vi "3_2_MNIST_Inference(FPGA)(PXI).vi"() -> ()   [LabVIEW 2020]
uses:
  <vilib>/userDefined/High Color/nirio_resource_hc.ctl
  <vilib>/Ngene/DeepLTK FPGA Addon/Toolkit/NNF_Host/Low_Level/NNF_Init/Controls/NNF_FPGA_Target_Info.ctl
  <extravilib>/ChannelInstances/Tag-bool/Write With Abort.vi
  <extravilib>/ChannelInstances/Tag-bool/Read With Abort.vi
  <extravilib>/ChannelInstances/Tag-bool/Instantiate.vi
  <vilib>/FPGAPlugInAG/Dynamic/niLvFpga_Download_Dynamic.vi
  <vilib>/FPGAPlugInAG/Dynamic/niLvFpga_Run_Dynamic.vi
  <extravilib>/ChannelInstances/Tag-bool/EndpointRead.vi
  <vilib>/Ngene/DeepLTK FPGA Addon/Toolkit/NNF_Host/API/NNF_Set_Input/NNF_Set_Input(2D_I8).vi
  <vilib>/FPGAPlugInAG/Dynamic/niLvFpga_Close_Dynamic.vi
  <extravilib>/ChannelInstances/Tag-bool/Endpoint.vi
  <vilib>/rvi/interface/nirviMethod/nirviMethod.xnode
  <vilib>/rvi/interface/nirviCloseFPGA/nirviCloseFPGA.xnode
  <extravilib>/ChannelInstances/Tag-bool.lvlib
  <vilib>/Ngene/DeepLTK FPGA Addon/Toolkit/DeepLTK_FPGA_Addon.lvlib
  <vilib>/Ngene/Deep Learning Toolkit/Toolkit/Deep_Learning_Toolkit_by_Ngene.lvlib
  <vilib>/ptbypt/NI_PtbyPt.lvlib
panel:
  out "Target Information":T1={"BRAM _Buff_1_Size"=52500, "BRAM _Buff_2_Size"=45937, "Version"=[8, 1, 1, 0], "# Cores"=8}
  out "Predictions":sgl[](array[slide])=[5.797983e-07, 2.833721e-05, 6.34908e-06, 0.999726, 5.797983e-07, 6.952559e-05, 3.4902146e-06, 1.1549668e-05, 9.3772185e-05, 5.9866026e-05] scale=0.0..1.0
  out "test time(s/img)":dbl=0.014425458999976399 format="%#_3p"
  out "Test Speed (img/s)":dbl=69.32188431589151 format="%#_3p"
  in  "FPGA Bitfile":path=path "D:/Ngene/GitHub/deepltk_fpga_examples/FPGA Bitfiles/NNF_sbRIO_9609_8Cores.lvbitx"
  in  "FPGA Target":T2="rio://10.0.0.39/RIO0" caption="RIO Device"
  in  "Weight File Path":path=path "D:/Ngene/GitHub/deepltk_fpga_examples/1_MNIST_Classification(PXI,sbRIO)/Models/1_Converted/mnist_cnn/NNF_mnist_cnn_weights_24_11_25__15_36_06.bin"
  in  "Configuration File Path":path=path "D:/Ngene/GitHub/deepltk_fpga_examples/1_MNIST_Classification(PXI,sbRIO)/Models/1_Converted/mnist_cnn/NNF_mnist_cnn_net_cfg_24_11_25__15_36_06.cfg"
  in  "Scalers File Path":path=path "D:/Ngene/GitHub/deepltk_fpga_examples/1_MNIST_Classification(PXI,sbRIO)/Models/1_Converted/mnist_cnn/NNF_mnist_cnn_net_scalers_24_11_25__15_36_06.cfg"
  out "Labels":string[](array[string])=["0", "1", "2", "3", "4", "5", "6", "7", "8", "9"]
  out "Pen Attributes":T3={"Width"=24, "Style"=enum."Solid"}
  out "Draw Digit (280x280 px)":picture
  in  "Pen Color":u32(colorbox)=197379
  in  "Stop":bool
  in  "Pen Width":dbl=24.0
  in  "Stop":bool
  out "image (28x28px)":sgl[][](graph)=[[-1.0, -1.0, -1.0, -1.0, -1.0, -1.0, -1.0, -1.0, -1.0, -1.0, -1.0, -1.0, -1.0, -1.0, -1.0, -1.0, -1.0, -1.0, -1.0, -1.0, -1.0, -1.0, -1.0, -1.0, -1.0, -1.0, -1.0, -1.0], [-1.0, -1.0, -1.0, -1.0, -1.0, -1.0, -1.0, -1.0, -1.0, -1.0, -1.0, -1.0, -1.0, -1.0, -1.0, -1.0, -1.0, -1.0, -1.0, -1.0, -1.0, -1.0, -1.0, -1.0, -1.0, -1.0, -1.0, -1.0], [-1.0, -1.0, -1.0, -1.0, -1.0, -1.0, -1.0, -0.96015626, -0.56171876, -0.1234375, 0.17539063, 0.49414062, 0.59375, 0.59375, 0.59375, 0.41445312, -0.08359375, -0.96015626, -1.0, -1.0, -1.0, -1.0, -1.0, -1.0, -1.0, -1.0, -1.0, -1.0], [-1.0, -1.0, -1.0, -1.0, -1.0, -0.9003906, 0.055859376, 0.8527344, 0.9921875, 0.9921875, 0.9921875, 0.9921875, 0.9921875, 0.9921875, 0.9921875, 0.9921875, 0.9921875, 0.6734375, -0.80078125, -1.0, -1.0, -1.0, -1.0, -1.0, -1.0, -1.0, -1.0, -1.0], [-1.0, -1.0, -1.0, -1.0, -0.840625, 0.77304685, 0.9921875, 0.9921875, 0.9921875, 0.9125, 0.6136719, 0.29492188, 0.1953125, 0.1953125, 0.1953125, 0.5738281, 0.9921875, 0.9921875, 0.17539063, -1.0, -1.0, -1.0, -1.0, -1.0, -1.0, -1.0, -1.0, -1.0], [-1.0, -1.0, -1.0, -1.0, -0.5816406, 0.9921875, 0.9921875, 0.37460938, -0.521875, -0.9800781, -1.0, -1.0, -1.0, -1.0, -1.0, -1.0, 0.7132813, 0.9921875, 0.31484374, -1.0, -1.0, -1.0, -1.0, -1.0, -1.0, -1.0, -1.0, -1.0], [-1.0, -1.0, -1.0, -1.0, -1.0, -0.22304687, -0.22304687, -1.0, -1.0, -1.0, -1.0, -1.0, -1.0, -1.0, -1.0, 0.095703125, 0.9921875, 0.9921875, 0.055859376, -1.0, -1.0, -1.0, -1.0, -1.0, -1.0, -1.0, -1.0, -1.0], [-1.0, -1.0, -1.0, -1.0, -1.0, -1.0, -1.0, -1.0, -1.0, -1.0, -1.0, -1.0, -1.0, -1.0, 0.095703125, 0.9921875, 0.9921875, 0.63359374, -0.80078125, -1.0, -1.0, -1.0, -1.0, -1.0, -1.0, -1.0, -1.0, -1.0], [-1.0, -1.0, -1.0, -1.0, -1.0, -1.0, -1.0, -1.0, -1.0, -1.0, -1.0, -1.0, -1.0, 0.095703125, 0.9921875, 0.9921875, 0.6734375, -0.80078125, -1.0, -1.0, -1.0, -1.0, -1.0, -1.0, -1.0, -1.0, -1.0, -1.0], [-1.0, -1.0, -1.0, -1.0, -1.0, -1.0, -1.0, -1.0, -1.0, -1.0, -1.0, -0.9203125, 0.37460938, 0.9921875, 0.9921875, 0.65351564, -0.80078125, -1.0, -1.0, -1.0, -1.0, -1.0, -1.0, -1.0, -1.0, -1.0, -1.0, -1.0], [-1.0, -1.0, -1.0, -1.0, -1.0, -1.0, -1.0, -1.0, -1.0, -0.68125, -0.1234375, 0.7332031, 0.9921875, 0.9921875, 0.9921875, 0.6734375, -0.14335938, -1.0, -1.0, -1.0, -1.0, -1.0, -1.0, -1.0, -1.0, -1.0, -1.0, -1.0], [-1.0, -1.0, -1.0, -1.0, -1.0, -1.0, -1.0, -1.0, 0.0359375, 0.9921875, 0.9921875, 0.9921875, 0.9921875, 0.9921875, 0.9921875, 0.9921875, 0.9921875, -0.023828125, -1.0, -1.0, -1.0, -1.0, -1.0, -1.0, -1.0, -1.0, -1.0, -1.0], [-1.0, -1.0, -1.0, -1.0, -1.0, -1.0, -1.0, -1.0, 0.753125, 0.9921875, 0.9921875, 0.79296875, 0.25507814, 0.055859376, 0.1953125, 0.7132813, 0.9921875, 0.8925781, -0.9003906, -1.0, -1.0, -1.0, -1.0, -1.0, -1.0, -1.0, -1.0, -1.0], [-1.0, -1.0, -1.0, -1.0, -1.0, -1.0, -1.0, -1.0, -0.521875, -0.00390625, -0.42226562, -0.9800781, -1.0, -1.0, -1.0, -0.16328125, 0.9921875, 0.9921875, -0.9203125, -1.0, -1.0, -1.0, -1.0, -1.0, -1.0, -1.0, -1.0, -1.0], [-1.0, -1.0, -1.0, -1.0, -1.0, -1.0, -1.0, -1.0, -1.0, -1.0, -1.0, -1.0, -1.0, -1.0, -1.0, -0.1234375, 0.9921875, 0.9921875, -1.0, -1.0, -1.0, -1.0, -1.0, -1.0, -1.0, -1.0, -1.0, -1.0], [-1.0, -1.0, -1.0, -1.0, -1.0, -1.0, -1.0, -1.0, -1.0, -1.0, -1.0, -1.0, -1.0, -1.0, -0.7609375, 0.8527344, 0.9921875, 0.79296875, -1.0, -1.0, -1.0, -1.0, -1.0, -1.0, -1.0, -1.0, -1.0, -1.0], [-1.0, -1.0, -1.0, -1.0, -1.0, -1.0, -1.0, -1.0, -1.0, -1.0, -1.0, -1.0, -1.0, -0.80078125, 0.6933594, 0.9921875, 0.9722656, -0.40234375, -1.0, -1.0, -1.0, -1.0, -1.0, -1.0, -1.0, -1.0, -1.0, -1.0], [-1.0, -1.0, -1.0, -1.0, -1.0, -1.0, -1.0, -1.0, -1.0, -1.0, -1.0, -1.0, -0.7210938, 0.6933594, 0.9921875, 0.9921875, -0.06367187, -1.0, -1.0, -1.0, -1.0, -1.0, -1.0, -1.0, -1.0, -1.0, -1.0, -1.0], [-1.0, -1.0, -1.0, -1.0, -1.0, -1.0, -1.0, -1.0, -1.0, -1.0, -0.9003906, -0.22304687, 0.8726562, 0.9921875, 0.9921875, 0.095703125, -1.0, -1.0, -1.0, -1.0, -1.0, -1.0, -1.0, -1.0, -1.0, -1.0, -1.0, -1.0], [-1.0, -1.0, -0.9800781, 0.275, 0.79296875, 0.79296875, 0.79296875, 0.79296875, 0.79296875, 0.8726562, 0.9921875, 0.9921875, 0.9921875, 0.9722656, -0.023828125, -1.0, -1.0, -1.0, -1.0, -1.0, -1.0, -1.0, -1.0, -1.0, -1.0, -1.0, -1.0, -1.0], [-1.0, -1.0, -0.840625, 0.9921875, 0.9921875, 0.9921875, 0.9921875, 0.9921875, 0.9921875, 0.9921875, 0.9921875, 0.9921875, 0.7332031, -0.6015625, -1.0, -1.0, -1.0, -1.0, -1.0, -1.0, -1.0, -1.0, -1.0, -1.0, -1.0, -1.0, -1.0, -1.0], [-1.0, -1.0, -1.0, -0.2828125, 0.17539063, 0.13554688, 0.0359375, 0.1953125, 0.095703125, -0.00390625, -0.203125, -0.6015625, -0.96015626, -1.0, -1.0, -1.0, -1.0, -1.0, -1.0, -1.0, -1.0, -1.0, -1.0, -1.0, -1.0, -1.0, -1.0, -1.0], [-1.0, -1.0, -1.0, -1.0, -1.0, -1.0, -1.0, -1.0, -1.0, -1.0, -1.0, -1.0, -1.0, -1.0, -1.0, -1.0, -1.0, -1.0, -1.0, -1.0, -1.0, -1.0, -1.0, -1.0, -1.0, -1.0, -1.0, -1.0], [-1.0, -1.0, -1.0, -1.0, -1.0, -1.0, -1.0, -1.0, -1.0, -1.0, -1.0, -1.0, -1.0, -1.0, -1.0, -1.0, -1.0, -1.0, -1.0, -1.0, -1.0, -1.0, -1.0, -1.0, -1.0, -1.0, -1.0, -1.0], [-1.0, -1.0, -1.0, -1.0, -1.0, -1.0, -1.0, -1.0, -1.0, -1.0, -1.0, -1.0, -1.0, -1.0, -1.0, -1.0, -1.0, -1.0, -1.0, -1.0, -1.0, -1.0, -1.0, -1.0, -1.0, -1.0, -1.0, -1.0], [-1.0, -1.0, -1.0, -1.0, -1.0, -1.0, -1.0, -1.0, -1.0, -1.0, -1.0, -1.0, -1.0, -1.0, -1.0, -1.0, -1.0, -1.0, -1.0, -1.0, -1.0, -1.0, -1.0, -1.0, -1.0, -1.0, -1.0, -1.0], [-1.0, -1.0, -1.0, -1.0, -1.0, -1.0, -1.0, -1.0, -1.0, -1.0, -1.0, -1.0, -1.0, -1.0, -1.0, -1.0, -1.0, -1.0, -1.0, -1.0, -1.0, -1.0, -1.0, -1.0, -1.0, -1.0, -1.0, -1.0], [-1.0, -1.0, -1.0, -1.0, -1.0, -1.0, -1.0, -1.0, -1.0, -1.0, -1.0, -1.0, -1.0, -1.0, -1.0, -1.0, -1.0, -1.0, -1.0, -1.0, -1.0, -1.0, -1.0, -1.0, -1.0, -1.0, -1.0, -1.0]]
  # "Overview: Demonstrates the usage of DeepLTK FPGA Addon for loading the model pretrained for MNIST Classification and running for inference on FPGA Targets in PXI sytems.\nRequirements:\n•DeepLTK - Deep Learning Toolkit for LabVIEW (https://www.ngene.co/deep-learning-toolkit-for-labview)\n•DeepLTK FPGA Addon (https://www.ngene.co/deepltk-accelerator-for-fpga)\nInstructions:\n1. Select FPGA target at FPGA Target control. PXI or remote sbRIO FPGA target can be specified.\n2. Provide path to compiled FPGA bitfile at FPGA Bitfile control.\n3. Provide paths to .cfg, .bin and scalers.cfg files generated during model conversion at Network Configuration File Path , Weight File Path  and Scalers File Path controls.\n4. Run the VI\n5.\tDraw a digit on the \"Draw Digit\" interface and observe the predictions results.\n6. Press the Stop button to stop the VI."
  # "Copy resource path from NI MAX if needed"
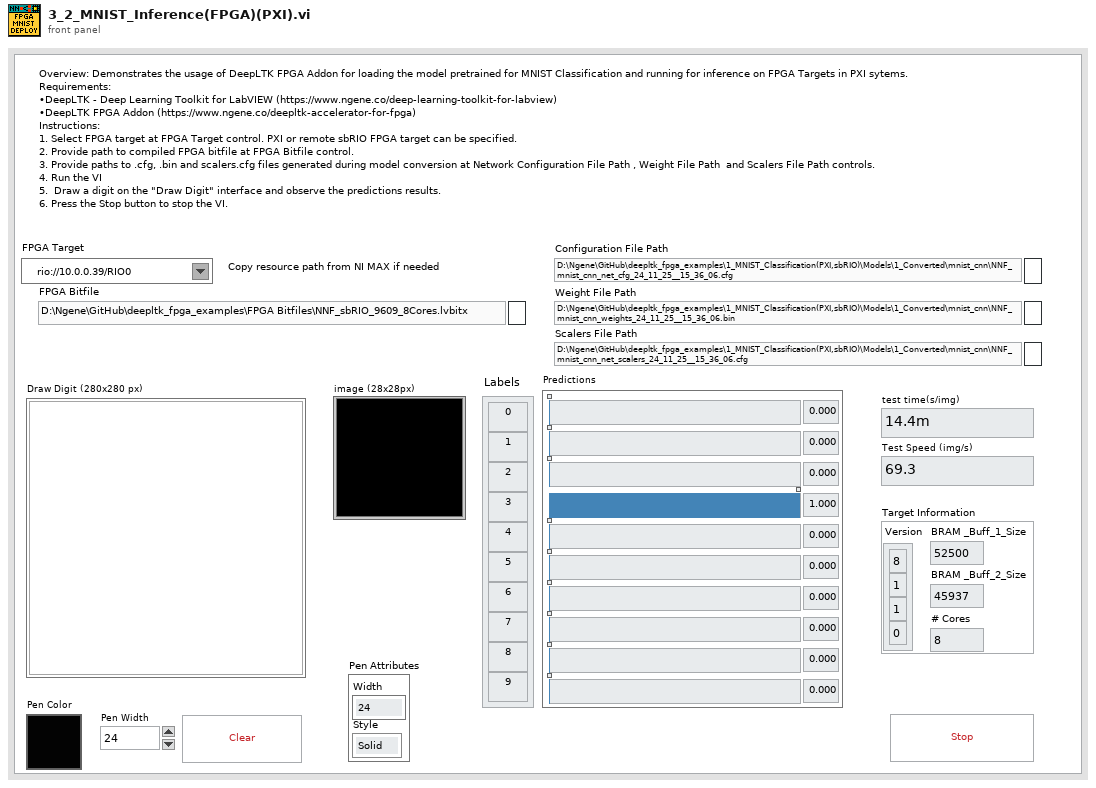
[diagram p1: front panel]
types:
  T1 = typedef "DeepLTK_FPGA_Addon.lvlib/NNF_FPGA_Target_Info.ctl" = cluster{"BRAM _Buff_1_Size":u32, "BRAM _Buff_2_Size":u32, "Version":u8[], "# Cores":u32}
  T2 = typedef "nirio_resource_hc.ctl" = tag
  T3 = cluster{"Width":u16, "Style":enum32{"Solid", "Dash", "Dot", "DashDot", "DashDotDot"}}
  T4 = typedef "DeepLTK_FPGA_Addon.lvlib/NNF.ctl" = cluster{"FPGA VI Ref ":refnum<k20>, "Subnets":T5[], "Dims_In":T7, "#Cores(enum)":T8, "NN_Ref":T9}
  T5 = typedef "DeepLTK_FPGA_Addon.lvlib/NNF_Subnet.ctl" = cluster{"Subnet Type":T6, "Subnet Data":variant, "Input Scaler":sgl, "Output Scaler":sgl}
  T6 = typedef "DeepLTK_FPGA_Addon.lvlib/NNF_Subnet_Type.ctl" = enum16{"CPU", "FPGA", "Split FPGA"}
  T7 = typedef "Deep_Learning_Toolkit_by_Ngene.lvlib/NN_Dims(C,H,W).ctl" = cluster{"C":i32, "H":i32, "W":i32}
  T8 = typedef "DeepLTK_FPGA_Addon.lvlib/NNF_No_Of_Cores.ctl" = enum16{"4CH", "8CH"}
  T9 = typedef "DeepLTK_FPGA_Addon.lvlib/NN_DVR.ctl" = refnum<data-value>
  T10 = cluster{"left":i16, "top":i16, "right":i16, "bottom":i16}
  T11 = typedef "LVMouseTypeDef.ctl" = cluster{"Mouse Position":cluster{"X":i32, "Y":i32}, "Mouse Modifiers":cluster{"Button Down":bool, "Shift Mod":bool, "Menu Mod":bool, "Option Mod":bool}}
  T12 = typedef "Tag-bool.lvlib/))Channel.ctl" = refnum<queue>
  T13 = typedef "imagedata.ctl" = cluster{"image type":i32, "image depth":i32, "image":u8[], "mask":u8[], "colors":u32[], "Rectangle":cluster{"left":i16, "top":i16, "right":i16, "bottom":i16}}
  T14 = typedef "Deep_Learning_Toolkit_by_Ngene.lvlib/NN_Layer.ctl" = cluster{"Name":string, "Layer_Data":variant, "Layer_Type":T15, "Dims_In":T7, "Layers_In":variant, "Dims_Out":T7, "Layers_Out":variant, "Metrics":T16, "GPU_Data":variant, "mBatch":i32, "NN_Device":T17, "NNg_hdls":T18, "Train?":bool, "Dimty":T19, "RecptField":T20}
  T15 = typedef "Deep_Learning_Toolkit_by_Ngene.lvlib/NN_Layer_Type.ctl" = enum16{"Input1D", "Input3D", "Conv1D", "Conv2D", "Conv2D_Adv", "MaxPool", "AvgPool", "UpSample", "DropOut3D", "ShortCut", "Concat", "SoftMax3D", "FC", "DropOut", "Softmax", "Flatten", "YOLO_v2", "YOLO_v4", "Activation", "BatchNormalization", "Unsupported"}
  T16 = typedef "Deep_Learning_Toolkit_by_Ngene.lvlib/NN_Layer_Metrics.ctl" = cluster{"Data":dbl, "Params":dbl, "Ops":dbl}
  T17 = typedef "Deep_Learning_Toolkit_by_Ngene.lvlib/NN_Device.ctl" = enum16{"CPU", "GPU"}
  T18 = typedef "Deep_Learning_Toolkit_by_Ngene.lvlib/nng_cuda_handles.ctl" = cluster{"cudnn":u64, "cublas":u64, "stream":u64, "curand":u64}
  T19 = typedef "Deep_Learning_Toolkit_by_Ngene.lvlib/NN_Layer_Dimty.ctl" = enum16{"1D", "3D"}
  T20 = typedef "Deep_Learning_Toolkit_by_Ngene.lvlib/NN_Layer_RF_State.ctl" = cluster{"Dims":T21, "J":T21}
  T21 = typedef "Deep_Learning_Toolkit_by_Ngene.lvlib/NN_Dims(V,H).ctl" = cluster{"V":i32, "H":i32}
  T22 = typedef "Deep_Learning_Toolkit_by_Ngene.lvlib/NN.ctl" = cluster{"Name":string, "No of Layers":i32, "mBatch":i32, "Layers":T23[], "Dimty":T24, "Dims_In":T7, "Dims_Out":T7, "Working_Dir":path, "Train?":bool, "Train_Params":T25, "LR_Update_Policy":T28, "Session Data":T30, "Ground_truth":T31, "NNg_hdls":T18, "NN_Device":T17, "GPU Id":i32, "Labels":string[], "Receptive Field":T21[], "Loss_Type":T32, "Loss_Cfg_Prms":variant, "NNG_WS":T33}
  T23 = typedef "Deep_Learning_Toolkit_by_Ngene.lvlib/NN_Layer_ref.ctl" = refnum<data-value>
  T24 = typedef "Deep_Learning_Toolkit_by_Ngene.lvlib/NN_In_Out_Dim-ty.ctl" = enum8{"In1D_Out1D", "In3D_Out1D", "In3D_Out3D", "In3D_OutBBox"}
  T25 = typedef "Deep_Learning_Toolkit_by_Ngene.lvlib/NN_Train_Params.ctl" = cluster{"Optimizer":T26, "Beta_1":sgl, "Beta_2":sgl, "Weight Decay(L1)":sgl, "Weight Decay(L2)":sgl, "Data_Sampling":T27}
  T26 = typedef "Deep_Learning_Toolkit_by_Ngene.lvlib/NN_Train_Optimizer.ctl" = enum16{"SGD", "Adam", "Adagrad", "Adadelta", "RMSProp", "Nesterov"}
  T27 = typedef "Deep_Learning_Toolkit_by_Ngene.lvlib/NN_Train_Data_Sampling.ctl" = enum16{"Random", "Sequential"}
  T28 = typedef "Deep_Learning_Toolkit_by_Ngene.lvlib/NN_LR_Policy_Cfg.ctl" = cluster{"Policy_Type":T29, "LR0":dbl, "k":sgl, "WarmUp_Policy":enum16{"Step", "Ramp"}, "WarmUp_Iter":i32, "WarmUp_Ratio":sgl}
  T29 = typedef "Deep_Learning_Toolkit_by_Ngene.lvlib/NN_LR_Policy_Type.ctl" = enum16{"Manual", "Step", "Exp", "1/t"}
  T30 = typedef "Deep_Learning_Toolkit_by_Ngene.lvlib/NN_Train_Session_Data.ctl" = cluster{"Epochs":sgl, "Tot_Iter":i32, "LR":sgl, "LR_iter":i32}
  T31 = typedef "Deep_Learning_Toolkit_by_Ngene.lvlib/NN_Ground_truth.ctl" = cluster{"Y":variant}
  T32 = typedef "Deep_Learning_Toolkit_by_Ngene.lvlib/NN_Loss_Type.ctl" = enum16{"None", "MSE", "CrossEntropy", "YOLO_v2", "YOLO_v4"}
  T33 = typedef "Deep_Learning_Toolkit_by_Ngene.lvlib/NNG_WS.ctl" = cluster{"NNG_WS_Mem":T34, "Max_WS_Size":i64}
  T34 = typedef "Deep_Learning_Toolkit_by_Ngene.lvlib/NNg_WS_Mem_DVR.ctl" = refnum<data-value>
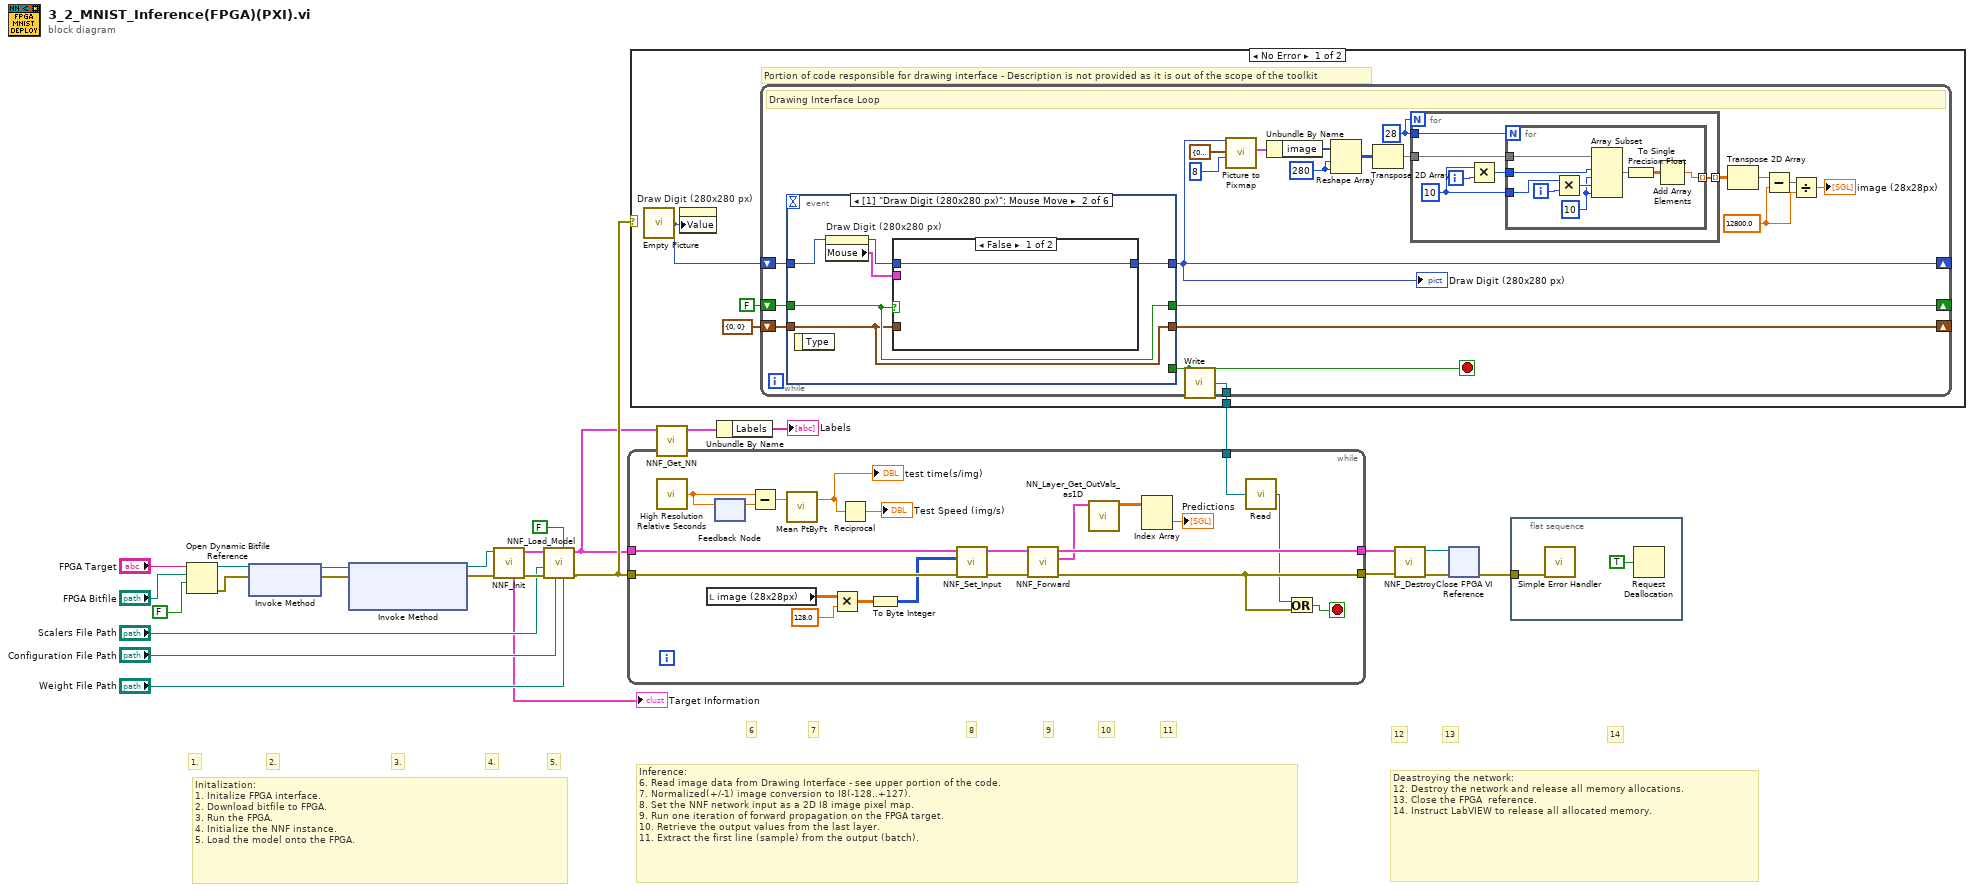
[diagram p0: block diagram]
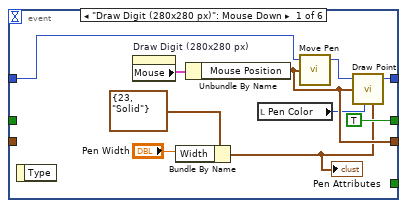
[diagram p2: hidden frame]
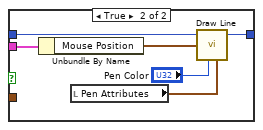
[diagram p3: hidden frame]
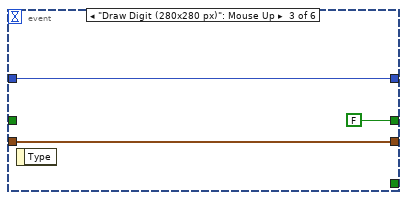
[diagram p4: hidden frame]
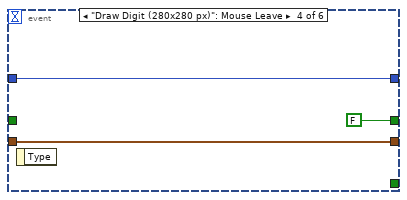
[diagram p5: hidden frame]
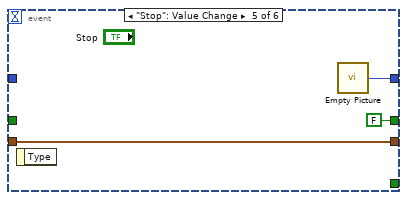
[diagram p6: hidden frame]
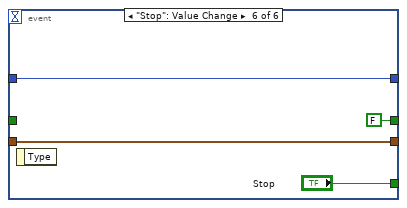
[diagram p7: hidden frame]
diagram:
  # "Deastroying the network:\n12. Destroy the network and release all memory allocations.\n13. Close the FPGA  reference.\n14. Instruct LabVIEW to release all allocated memory."
  # "14"
  # "13"
  # "12"
  # "11"
  # "10"
  # "9"
  # "8"
  # "7"
  # "6"
  # "Inference:\n6. Read image data from Drawing Interface - see upper portion of the code.\n7. Normalized(+/-1) image conversion to I8(-128..+127).\n8. Set the NNF network input as a 2D I8 image pixel map.\n9. Run one iteration of forward propagation on the FPGA target.\n10. Retrieve the output values from the last layer.\n11. Extract the first line (sample) from the output (batch)."
  # "5."
  # "Initalization:\n1. Initalize FPGA interface.\n2. Download bitfile to FPGA.\n3. Run the FPGA.\n4. Initialize the NNF instance.\n5. Load the model onto the FPGA."
  # "4."
  # "3."
  # "2."
  # "1."
  n1 = Open Dynamic Bitfile Reference(0:"FPGA Target", 1:"FPGA Bitfile", 2:FALSE ("Run When Loaded")) -> (5:w18:refnum<k20>, 8:w16:errorcluster)  [unwired: 2 in]
  n2 = xnode "Invoke Method"("FPGA VI Reference In"=w18, "error in"=w16) -> ("FPGA VI Reference Out"=w17:refnum<k20>, "error out"=w15:errorcluster)
  n3 = xnode "Invoke Method"("FPGA VI Reference In"=w17, "error in"=w15) -> ("FPGA VI Reference Out"=w20:refnum<k20>, "error out"=w23:errorcluster)  [unwired: 1 in]
  n4 = call <vilib>:"NNF_Init.vi"("error in"=w23, "FPGA Interface"=w20) -> ("error out"=w26:errorcluster, "NNF out"=w25:T4, "Target Information"=→"Target Information":T1)  [unwired: 7 in]
  n5 = call <vilib>:"NNF_Load_Model.vi"("Weight File Path"="Weight File Path", "Force CPU(All)?"=FALSE, "Network CFG File Path"="Configuration File Path", "Error in"=w26, "Scalers"="Scalers File Path", "NNF in"=w25) -> ("error Out"=w11:errorcluster, "NNF out"=w10:T4)  [unwired: 4 in]
  n6 = case shown="No Error" w11 {
    tunnel: [w27 _] -> w9
    frame No Error {
      # "Portion of code responsible for drawing interface - Description is not provided as it is out of the scope of the toolkit"
      n7 = call "Empty Picture"() -> ("empty picture"=w30:picture)
      n8 = property on="Draw Digit (280x280 px)" class="Pict"("Value"=w30) -> ()  [unwired: 2 in, 2 out]
      n9 = while {
        shift-right: [w46] -> _
        shift-left: w30 -> [w51]
        shift-right: [w49] -> _
        shift-left: FALSE -> [w50]
        shift-right: [w47] -> _
        shift-left: cluster{"X":i32, "Y":i32} {"X"=0, "Y"=0} ("Mouse Position") -> [w48]
        tunnel: [w33] -> w27
        stop <- w38 stop-if-true
        w35 = sgl 12800.0 ("dimension size")
        w39 = 280 ("dimension size")
        w41 = 28
        # "Drawing Interface Loop"
        n10 = event shown="[1] \"Draw Digit (280x280 px)\": Mouse Move" {
          selector: _ -> [_ _ _ _ _ _]
          dyn-events: _ -> [_ _ _ _ _ _]
          timeout: _ -> [_ _ _ _ _ _]
          tunnel: [_ _ _ _ _ "Stop"] -> w38
          tunnel: [w73 w80 w91 w94 w97 w100] -> w46
          tunnel: w51 -> [w75 w79 w91 w94 _ w100]
          tunnel: w50 -> [_ w78 _ _ _ _]
          tunnel: [TRUE w78 FALSE FALSE FALSE FALSE] -> w49
          tunnel: w48 -> [_ w77 w89 w93 w96 w99]
          tunnel: [w71 w77 w89 w93 w96 w99] -> w47
          event "Draw Digit (280x280 px)": Mouse Down {
            # "Set the pen position, and draw an initial point or line."
            n11 = event-data() -> ()  [unwired: 1 in, 1 out]
            n12 = property on="Draw Digit (280x280 px)" class="Pict"() -> ("Mouse"=w76:T11)  [unwired: 2 in, 2 out]
            n13 = Bundle By Name(cluster=T3 {"Width"=23, "Style"=enum."Solid"} ("Pen Attributes"), "Width"="Pen Width") -> (w67:T3)
            "Pen Attributes" <- w67
            n14 = Unbundle By Name(w76) -> ("Mouse Position"=w71:cluster{"X":i32, "Y":i32})
            n15 = local read "Pen Color"() -> (w70:u32)
            n16 = call <vilib>:"Move Pen.vi"("new position"=w71, "picture"=w75) -> ("new picture"=w74:picture)  [unwired: 3 in]
            n17 = call <vilib>:"Draw Point.vi"("picture"=w74, "point(x,y)"=w71, "color(black)"=w70, "pen"=w67) -> ("new picture"=w73:picture)  [unwired: 5 in]
          }
          event "Draw Digit (280x280 px)": Mouse Move {
            # "Only draw if a Mouse Down event has occurred, but not a Mouse Up. Then, determine if the user is Drawing a point, a line, or selecting a subset and perform those operations in the case structure."
            n18 = event-data() -> ()  [unwired: 1 in, 1 out]
            n19 = property on="Draw Digit (280x280 px)" class="Pict"() -> ("Mouse"=w81:T11)  [unwired: 2 in, 2 out]
            n20 = case shown="False" w78 {
              tunnel: w79 -> [w82 w88]
              tunnel: w81 -> [_ w87]
              tunnel: [w82 w85] -> w80
              tunnel: w77 -> [_ _]
              frame False {
              }
              frame True {
                n21 = Unbundle By Name(w87) -> ("Mouse Position"=w86:cluster{"X":i32, "Y":i32})
                n22 = local read "Pen Attributes"() -> (w84:T3)
                n23 = call <vilib>:"Draw Line.vi"("picture"=w88, "end point"=w86, "color(black)"="Pen Color", "pen"=w84) -> ("new picture"=w85:picture)  [unwired: 5 in]
              }
            }
          }
          event "Draw Digit (280x280 px)": Mouse Up {
            # "When the user is finished drawing, we complete the operation. The only operation that we need to complete the Select Subset operation."
            n24 = event-data() -> ()  [unwired: 1 in, 1 out]
          }
          event "Draw Digit (280x280 px)": Mouse Leave {
            # "Change to the default cursor when the mouse leaves the picture."
            n25 = event-data() -> ()  [unwired: 1 in, 1 out]
          }
          event "Stop": Value Change {
            # "Erase the picture."
            n26 = event-data() -> ()  [unwired: 1 in, 1 out]
            n27 = call "Empty Picture"() -> ("empty picture"=w97:picture)
          }
          event "Stop": Value Change {
            # "Stop the VI."
            n28 = event-data() -> ()  [unwired: 1 in, 1 out]
          }
        }
        "Draw Digit (280x280 px)" <- w46
        n29 = call <extravilib>:"Write.vi"("element"=w38) -> ("channel"=w33:T12)  [unwired: 1 out]
        n30 = call <vilib>:"Picture to Pixmap.vi"("depth"=8, "rect"=T10 {"left"=0, "top"=0, "right"=280, "bottom"=280}, "picture"=w46) -> ("image data"=w45:T13)  [unwired: 7 in, 1 out]
        n31 = Unbundle By Name(w45) -> ("image"=w44:u8[])
        n32 = Reshape Array(w44, w39, w39) -> (w43:u8[][])
        n33 = Transpose 2D Array(2D array=w43) -> (transposed array=w42:u8[][])
        n34 = for {
          N: w41 -> [_]
          tunnel: w42 -> [w57]
          tunnel: w41 -> [w56]
          tunnel: [w52] -> w40 mode=indexing
          i -> [w55]
          w53 = 10 ("x")
          n35 = Multiply(x=w53, y=w55) -> (x*y=w54:i32)
          n36 = for {
            N: w56 -> [_]
            tunnel: w57 -> [w66]
            tunnel: w54 -> [w65]
            tunnel: w53 -> [w62]
            tunnel: [w58] -> w52 mode=indexing
            i -> [w64]
            w61 = 10 ("length")
            n37 = Multiply(x=w62, y=w64) -> (x*y=w63:i32)
            n38 = Array Subset(array=w66, index (row)=w65, length (row)=w61, index (col)=w63, length (col)=w61) -> (w60:u8[][])
            n39 = To Single Precision Float(number=w60) -> (single precision float=w59:sgl[][])
            n40 = Add Array Elements(numeric array=w59) -> (sum=w58:sgl)
          }
        }
        n41 = Transpose 2D Array(2D array=w40) -> (transposed array=w36:sgl[][])
        n42 = Subtract(x=w36, y=w35) -> (x-y=w37:sgl[][])
        n43 = Divide(x=w37, y=w35) -> (x/y=→"image (28x28px)":sgl[][])
      }
    }
    frame Error {
    }
  }
  n44 = while {
    tunnel: w10 -> [w122]
    tunnel: w11 -> [w121]
    tunnel: [w118] -> w8
    tunnel: [w117] -> w5
    tunnel: w9 -> [w103]
    stop <- w116 stop-if-true
    n45 = call <vilib>:"High Resolution Relative Seconds.vi"() -> ("relative seconds"=w120:dbl)
    n46 = local read "image (28x28px)"() -> (w104:sgl[][])
    n47 = feedback #1() -> (w119:dbl)  [unwired: 1 in]
    n48 = feedback-in #1(w120) -> ()
    n49 = Subtract(x=w120, y=w119) -> (x-y=w107:dbl)
    n50 = call <vilib>:"Mean PtByPt.vi"("x"=w107) -> ("mean"=w106:dbl)  [unwired: 3 in, 1 out]
    "test time(s/img)" <- w106
    n51 = Multiply(x=w104, y=sgl 128.0 ("x")) -> (x*y=w111:sgl[][])
    n52 = Reciprocal(x=w106) -> (1/x=→"Test Speed (img/s)":dbl)
    n53 = To Byte Integer(number=w111) -> (8bit integer=w109:i8[][])
    n54 = call-poly <vilib>:"NNF_Set_Input.vi"("error in"=w121, "Data_in(2D_I8)"=w109, "NNF In"=w122) -> ("error out"=w112:errorcluster, "NNF out"=w113:T4)  [unwired: 7 in]
    n55 = call <vilib>:"NNF_Forward.vi"("error in"=w112, "NNF in"=w113) -> ("error out"=w117:errorcluster, "Last_Layer"=w115:T14, "NNF out"=w118:T4)  [unwired: 7 in]
    n56 = call <vilib>:"NN_Layer_Get_OutVals_as1D.vi"("Layer"=w115) -> ("Out(as1D)"=w114:sgl[][])  [unwired: 9 in, 1 out]
    n57 = Index Array(array=w114) -> (element=→"Predictions":sgl[])  [unwired: 2 in]
    n58 = call <extravilib>:"Read.vi"("channel"=w103) -> ("element"=w102:bool)  [unwired: 1 in, 1 out]
    n59 = Or(x=w102, y=w117) -> (x .or. y?=w116:bool)
  }
  n60 = call "NNF_Get_NN.vi"("NNF in"=w10) -> ("NN out"=w7:T22)  [unwired: 10 in]
  n61 = Unbundle By Name(w7) -> ("Labels"=→"Labels":string[])
  n62 = call <vilib>:"NNF_Destroy.vi"("error in"=w5, "NNF in"=w8) -> ("error out"=w2:errorcluster, "FPGA VI Ref"=w3:refnum<k20>)  [unwired: 8 in]
  n63 = xnode "Close FPGA VI Reference"("FPGA VI Reference In"=w3, "error in"=w2) -> ("error out"=w1:errorcluster)
  n64 = flat-sequence {
    tunnel: w1 -> [w124]
    frame #0 {
      n65 = call <vilib>:"Simple Error Handler.vi"("error in (no error)"=w124) -> ()  [unwired: 4 in, 5 out]
      n66 = Request Deallocation(TRUE ("flag")) -> ()
    }
  }
